vi "Frequency Analysis of a Filter Design.vi"() -> ()   [LabVIEW 2020]
doc: "Demonstrates how to test the frequency response of a digital filter against arbitrary specifications. This example uses a white noise signal as the stimulus of the filter, measures the frequency response between this stimulus and the response of the filter, and then tests if the result falls within some arbitrary limits. Various design parameters of the filter can be changed to successfully design the filter."
uses:
  <vilib>/Analysis/4window.llb/windowTd.ctl
  <vilib>/measure/mamon.llb/Create Continuous Mask.vi
  <vilib>/measure/macond.llb/IIR Filter for 1 Chan.vi
  <vilib>/measure/maspectr.llb/Frequency Response Function (Mag-Phase) 1-1.vi
  <vilib>/measure/mamon.llb/Limit Testing Frequency.vi
  <vilib>/measure/NI_MABase.lvlib
  <vilib>/measure/NI_MAPro.lvlib
  <vilib>/Analysis/NI_AALPro.lvlib
panel:
  in  "Upper Fc":dbl=3800.0
  in  "Lower Fc":dbl=2000.0
  in  "Order":i32=6
  in  "Stop":bool
  out "Passed?":bool
  out "Frequency Response":cluster{"x0":dbl, "dx":dbl, "Y":dbl[]}[](graph)
  # "Overview: Demonstrates how to test the frequency response of a digital filter against arbitrary specifications.\nRequirements: LabVIEW Full Development System\nInstructions:\n1. Run the VI.\n2. Change the IIR Filter Specifications to cause the Filter signal to pass the limit specifications.\n3. Click Stop to stop the VI."
  # "IIR Filter Specifications"
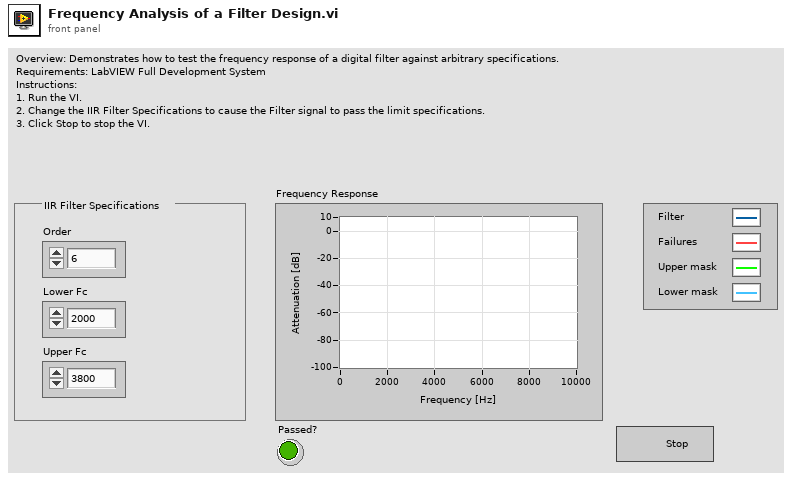
[diagram p1: front panel]
types:
  T1 = enum16{"No averaging", "Vector averaging", "RMS averaging", "Peak hold"}
  T2 = typedef "NI_AALPro.lvlib/windowTd.ctl" = u32
  T3 = cluster{"Topology":enum16{"Off", "Butterworth", "Chebyshev", "Inverse Chebyshev", "Elliptic", "Bessel"}, "Type":enum16{"Lowpass", "Highpass", "Bandpass", "Bandstop"}, "Order":i32, "Lower Fc":dbl, "Upper Fc":dbl, "PB Ripple":dbl, "SB Attenuation":dbl}
  T4 = cluster{"averaging mode":enum16{"No averaging", "Vector averaging", "RMS averaging", "Peak hold"}, "weighting mode":enum16{"Linear", "Exponential"}, "number of averages":u32}
  T5 = cluster{"dB On (F)":bool, "unwrap phase (F)":bool, "convert to degree (F)":bool}
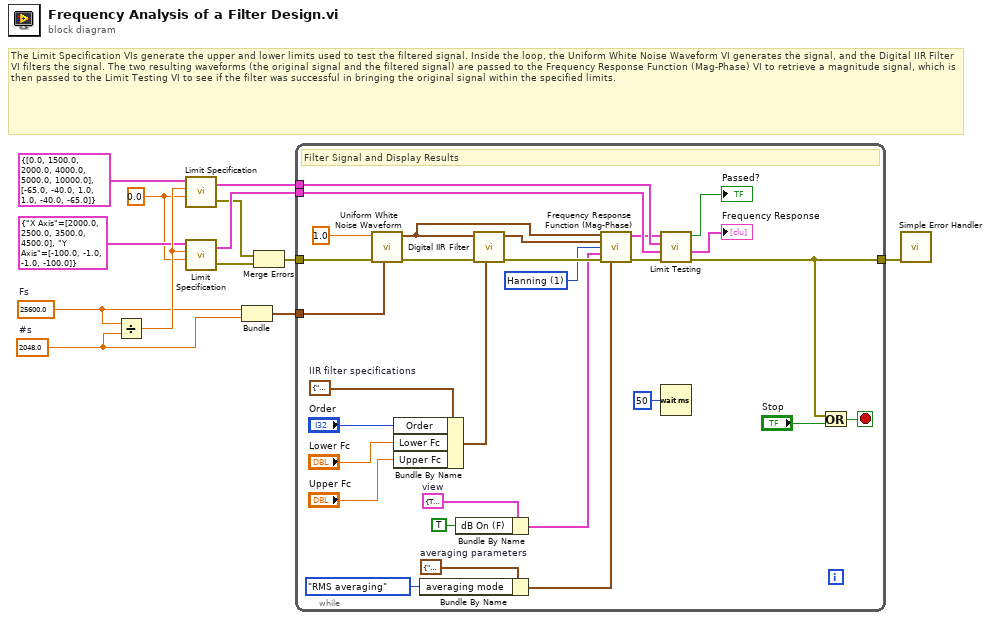
[diagram p0: block diagram]
diagram:
  w8 = 0.0
  w1 = 2048.0  # #s
  w2 = 25600.0  # Fs
  # "The Limit Specification VIs generate the upper and lower limits used to test the filtered signal. Inside the loop, the Uniform White Noise Waveform VI generates the signal, and the Digital IIR Filter VI filters the signal. The two resulting waveforms (the original signal and the filtered signal) are passed to the Frequency Response Function (Mag-Phase) VI to retrieve a magnitude signal, which is then passed to the Limit Testing VI to see if the filter was successful in bringing the original signal within the specified limits."
  n1 = Divide(x=w2, y=w1) -> (x/y=w12:dbl)
  n2 = call-poly <vilib>:"Limit Specification.vi"("Specification Cluster"=cluster{dbl[], dbl[]} {[0.0, 1500.0, 2000.0, 4000.0, 5000.0, 10000.0], [-65.0, -40.0, 1.0, 1.0, -40.0, -65.0]} ("Output Cluster"), "dx"=w12, "x0"=w8) -> ("Limit"=w11:cluster{"x0":dbl, "dx":dbl, "Y":dbl[]}, "error out"=w3:errorcluster)  [unwired: 2 in]
  n3 = call-poly <vilib>:"Limit Specification.vi"("Specification Cluster"=cluster{"X Axis":dbl[], "Y Axis":dbl[]} {"X Axis"=[2000.0, 2500.0, 3500.0, 4500.0], "Y Axis"=[-100.0, -1.0, -1.0, -100.0]}, "dx"=w12, "x0"=w8) -> ("Limit"=w6:cluster{"x0":dbl, "dx":dbl, "Y":dbl[]}, "error out"=w5:errorcluster)  [unwired: 2 in]
  n4 = Bundle("Fs"=w2, "#s"=w1) -> (w13:cluster{"Fs":dbl, "#s":dbl})  [unwired: 1 in]
  n5 = Merge Errors(w3, w5) -> (w4:errorcluster)
  n6 = while {
    tunnel: w6 -> [w38]
    tunnel: w11 -> [w39]
    tunnel: w13 -> [w40]
    tunnel: [w29] -> w7
    tunnel: w4 -> [w27]
    stop <- w30 stop-if-true
    w15 = T2 1 items=["Rectangle"=0, "Hanning"=1, "Hamming"=2, "Blackman-Harris"=3, "Exact Blackman"=4, "Blackman"=5, "Flat Top"=6, "4 Term B-Harris "=7, "7 Term B-Harris"=8, "Low Sidelobe"=9, "Blackman Nuttall"=11, "Triangle"=30, "Bartlett-Hanning"=31, "Bohman"=32, "Parzen"=33, "Welch"=34, "Kaiser"=60, "Dolph-Chebyshev"=61, "Gaussian"=62] ("window")
    w20 = T3 {"Topology"=enum."Butterworth", "Type"=enum."Bandpass", "Order"=7, "Lower Fc"=2000.0, "Upper Fc"=3800.0, "PB Ripple"=0.025, "SB Attenuation"=90.0}  # IIR filter specifications
    w21 = T4 {"averaging mode"=enum."RMS averaging", "weighting mode"=enum."Exponential", "number of averages"=10}  # averaging parameters
    w24 = T5 {"dB On (F)"=TRUE, "unwrap phase (F)"=FALSE, "convert to degree (F)"=FALSE}  # view
    # "Filter Signal and Display Results"
    n7 = call <vilib>:"Uniform White Noise Waveform.vi"("sampling info"=w40, "error in (no error)"=w27, "amplitude"=1.0) -> ("error out"=w33:errorcluster, "signal out"=w28:waveform(dbl))  [unwired: 7 in]
    n8 = Bundle By Name(cluster=w20, "Order"="Order", "Lower Fc"="Lower Fc", "Upper Fc"="Upper Fc") -> (w16:T3)
    n9 = Bundle By Name(cluster=w21, "averaging mode"=T1."RMS averaging") -> (w25:T4)
    n10 = Bundle By Name(cluster=w24, "dB On (F)"=TRUE) -> (w23:T5)
    n11 = call-poly <vilib>:"Digital IIR Filter.vi"("IIR filter specifications"=w16, "error in (no error)"=w33, "signal in"=w28) -> ("error out"=w41:errorcluster, "signal out"=w42:waveform(dbl))  [unwired: 6 in, 1 out]
    n12 = call-poly <vilib>:"Frequency Response Function (Mag-Phase).vi"("time signal X"=w28, "time signal Y"=w42, "window"=w15, "view"=w23, "error in (no error)"=w41, "averaging parameters"=w25) -> ("magnitude"=w35:cluster{"f0":dbl, "df":dbl, "magnitude":dbl[]}, "error out"=w32:errorcluster)  [unwired: 4 in, 4 out]
    n13 = call-poly <vilib>:"Limit Testing.vi"("error in (no error)"=w32, "lower limit"=w38, "upper limit"=w39, "signal in"=w35) -> ("error out"=w29:errorcluster, "output values"=→"Frequency Response":cluster{"x0":dbl, "dx":dbl, "Y":dbl[]}[], "test passed?"=→"Passed?":bool)  [unwired: 2 in, 3 out]
    n14 = Wait (ms)(milliseconds to wait=u32 50) -> ()  [unwired: 1 out]
    n15 = Or(x=w29, y="Stop") -> (x .or. y?=w30:bool)
  }
  n16 = call <vilib>:"Simple Error Handler.vi"("error in (no error)"=w7) -> ()  [unwired: 4 in, 5 out]
